vi "SVT Running RMS Level.vi"   [LabVIEW 2017]
doc: "Computes the running root-mean-square (RMS) level of <B>scaled signal [EU]</B>. <B>integration time [s]</B> specifies the duration over which the RMS level is computed. You can use this polymorphic VI to compute the running RMS level for a single channel or for N channels. The data type you wire to the <B>scaled signal [EU]</B> input determines the polymorphic instance to use."
uses:
  <vilib>/addons/Sound and Vibration/svt_Level/SoundVib_VibrationLevel.lvlib
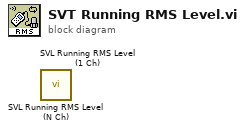
[diagram p0: block diagram]
diagram:
  n1 = call <vilib>:"SVL Running RMS Level (N Ch).vi"() -> ()  [unwired: 8 in, 4 out]
  n2 = call <vilib>:"SVL Running RMS Level (1 Ch).vi"() -> ()  [unwired: 8 in, 4 out]
